vi "New TDMS Property.vi"(8 "error in (no error)":errorcluster, 11 "TDMS Property":T1) -> (0 "error out":errorcluster, 3 "TDMSProperty Ref":T2)   [LabVIEW 2020, in "NI_VS Data Logging API.lvlib"]
doc: "Creates a TdmsProperty object based on the <b>TDMS Property</b> input. The values of TDMS properties that you add to the file, channel groups, or channels, must be scalars of one of the following data types: Timestamp, I8, I16, I32, I64, U8, U16, U32, U64, Single, Double, Boolean, or String. If you set the value to any other data type, or an array of any type, an error will occur."
uses:
  <vilib>/NI VeriStand/Execution/DataLogging/NI_VS Data Logging API.lvlib
  <vilib>/NI VeriStand/Execution/DataLogging/TdmsProperty Ref.ctl
  NationalInstruments.VeriStand.ClientAPI
  <vilib>/NI VeriStand/Execution/DataLogging/TDMS Property.ctl
  <vilib>/NI VeriStand/Execution/DataLogging/Constants.vi
  <vilib>/Utility/VariantDataType/VariantType.lvlib
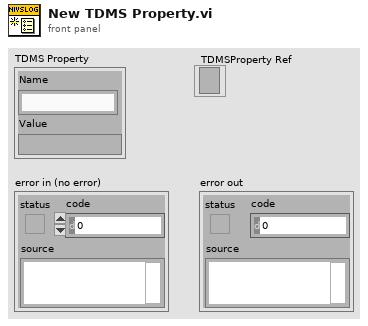
[diagram p1: front panel]
types:
  T1 = typedef "NI_VS Data Logging API.lvlib/TDMS Property.ctl" = cluster{"Name":string, "Value":variant}
  T2 = typedef "NI_VS Data Logging API.lvlib/TdmsProperty Ref.ctl" = refnum<k24>
  T3 = typedef "VariantType.lvlib/Type.ctl" = enum8{"Invalid Type", "Void", "I8", "I16", "I32", "I64", "U8", "U16", "U32", "U64", "Single Float", "Double Float", "Extended Float", "Single Complex", "Double Complex", "Extended Complex", "Enum U8", "Enum U16", "Enum U32", "Enum U64", "Single Float With Unit", "Double Float With Unit", "Extended Float With Unit", "Single Complex with Unit", "Double Complex with Unit", "Extended Complex with Unit", "Boolean", "String", "Path", "Picture", "Tag", "Array", "Cluster", "Variant", "LV Variant", "Waveform", "Timestamp", "Digital Waveform", "Digital Data", "ExpressData", "Refnum", "External Data", "VI", "Poly VI", "LabVIEW Class Instance", "Fixed Point"}
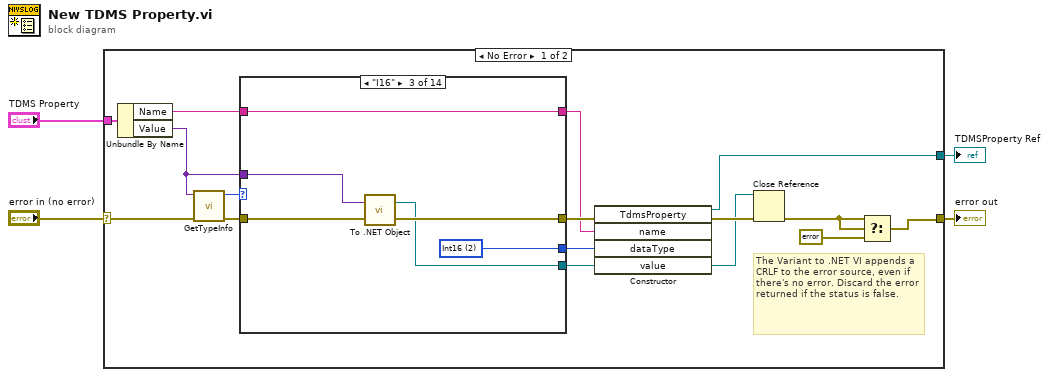
[diagram p0: block diagram]
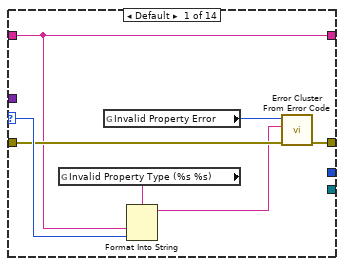
[diagram p2: hidden frame]
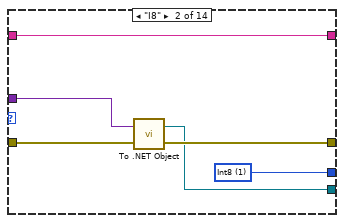
[diagram p3: hidden frame]
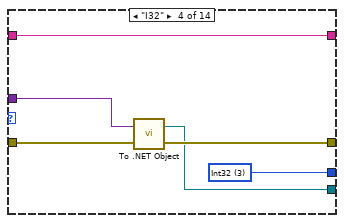
[diagram p4: hidden frame]
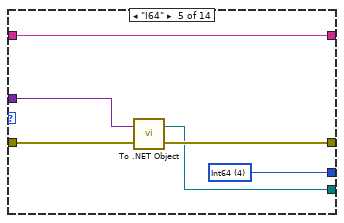
[diagram p5: hidden frame]
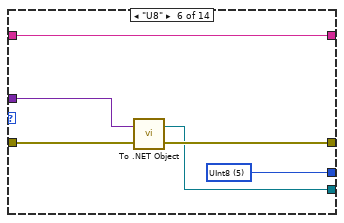
[diagram p6: hidden frame]
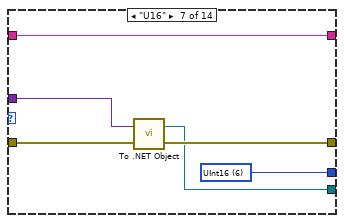
[diagram p7: hidden frame]
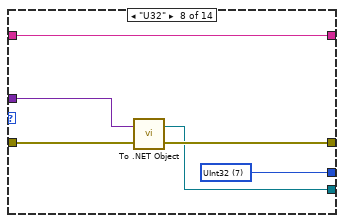
[diagram p8: hidden frame]
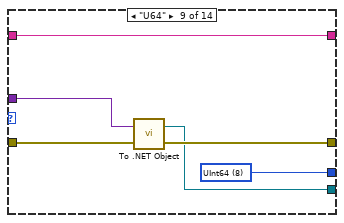
[diagram p9: hidden frame]
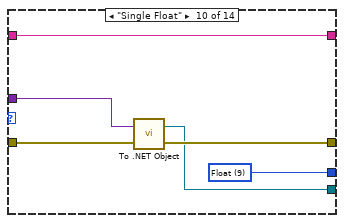
[diagram p10: hidden frame]
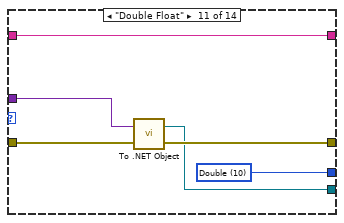
[diagram p11: hidden frame]
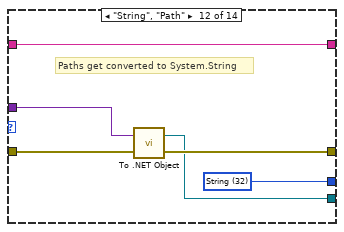
[diagram p12: hidden frame]
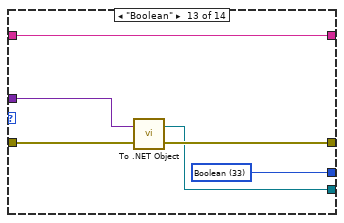
[diagram p13: hidden frame]
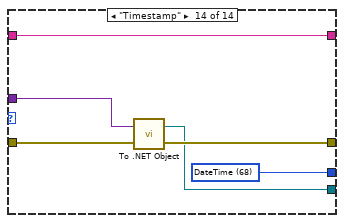
[diagram p14: hidden frame]
diagram:
  n1 = case shown="No Error" "error in (no error)" {
    selector: "error in (no error)" -> [w12 w105]
    tunnel: [w5 w105] -> w4
    tunnel: [w18 _] -> w3
    tunnel: "TDMS Property" -> [w13 _]
    frame No Error {
      # "The Variant to .NET VI appends a CRLF to the error source, even if there's no error. Discard the error returned if the status is false."
      n2 = Unbundle By Name(w13) -> ("Name"=w8:string, "Value"=w16:variant)
      n3 = call <vilib>:"GetTypeInfo.vi"("error in (no error)"=w12, "Variant"=w16) -> ("error out"=w15:errorcluster, "Type Enum"=w14:T3)  [unwired: 5 in, 3 out]
      n4 = case shown="\"I16\"" w14 {
        selector: w14 -> [w26 _ _ _ _ _ _ _ _ _ _ _ _ _]
        tunnel: w15 -> [w25 w31 w37 w43 w49 w55 w61 w67 w73 w79 w85 w91 w97 w103]
        tunnel: w16 -> [_ w30 w36 w42 w48 w54 w60 w66 w72 w78 w84 w90 w96 w102]
        tunnel: [_ w32 w38 w44 w50 w56 w62 w68 w74 w80 w86 w92 w98 w104] -> w17
        tunnel: [w24 w29 w35 w41 w47 w53 w59 w65 w71 w77 w83 w89 w95 w101] -> w19
        tunnel: [_ w28 w34 w40 w46 w52 w58 w64 w70 w76 w82 w88 w94 w100] -> w10
        tunnel: [w20 w27 w33 w39 w45 w51 w57 w63 w69 w75 w81 w87 w93 w99] -> w9
        tunnel: w8 -> [w20 w27 w33 w39 w45 w51 w57 w63 w69 w75 w81 w87 w93 w99]
        frame Default {
          n5 = global read "Constants.vi" "Invalid Property Type (%s %s)"() -> (w23:string)
          n6 = global read "Constants.vi" "Invalid Property Error"() -> (w21:i32)
          n7 = Format Into String(format string=w23, w20, w26) -> (resulting string=w22:string)  [unwired: 2 in, 1 out]
          n8 = call <vilib>:"Error Cluster From Error Code.vi"("error in (no error)"=w25, "error message (\"\")"=w22, "error code (0)"=w21) -> ("error out"=w24:errorcluster)  [unwired: 6 in]
        }
        frame "I8" {
          w32 = 1 items=["Int8"=1, "Int16"=2, "Int32"=3, "Int64"=4, "UInt8"=5, "UInt16"=6, "UInt32"=7, "UInt64"=8, "Float"=9, "Double"=10, "String"=32, "Boolean"=33, "DateTime"=68] ("dataType")
          n9 = call <vilib>:"To .NET Object.vi"("error in (no error)"=w31, "anything"=w30) -> ("error out"=w29:errorcluster, ".NET object"=w28:refnum<k24>)
        }
        frame "I16" {
          w38 = 2 items=["Int8"=1, "Int16"=2, "Int32"=3, "Int64"=4, "UInt8"=5, "UInt16"=6, "UInt32"=7, "UInt64"=8, "Float"=9, "Double"=10, "String"=32, "Boolean"=33, "DateTime"=68] ("dataType")
          n10 = call <vilib>:"To .NET Object.vi"("error in (no error)"=w37, "anything"=w36) -> ("error out"=w35:errorcluster, ".NET object"=w34:refnum<k24>)
        }
        frame "I32" {
          w44 = 3 items=["Int8"=1, "Int16"=2, "Int32"=3, "Int64"=4, "UInt8"=5, "UInt16"=6, "UInt32"=7, "UInt64"=8, "Float"=9, "Double"=10, "String"=32, "Boolean"=33, "DateTime"=68] ("dataType")
          n11 = call <vilib>:"To .NET Object.vi"("error in (no error)"=w43, "anything"=w42) -> ("error out"=w41:errorcluster, ".NET object"=w40:refnum<k24>)
        }
        frame "I64" {
          w50 = 4 items=["Int8"=1, "Int16"=2, "Int32"=3, "Int64"=4, "UInt8"=5, "UInt16"=6, "UInt32"=7, "UInt64"=8, "Float"=9, "Double"=10, "String"=32, "Boolean"=33, "DateTime"=68] ("dataType")
          n12 = call <vilib>:"To .NET Object.vi"("error in (no error)"=w49, "anything"=w48) -> ("error out"=w47:errorcluster, ".NET object"=w46:refnum<k24>)
        }
        frame "U8" {
          w56 = 5 items=["Int8"=1, "Int16"=2, "Int32"=3, "Int64"=4, "UInt8"=5, "UInt16"=6, "UInt32"=7, "UInt64"=8, "Float"=9, "Double"=10, "String"=32, "Boolean"=33, "DateTime"=68] ("dataType")
          n13 = call <vilib>:"To .NET Object.vi"("error in (no error)"=w55, "anything"=w54) -> ("error out"=w53:errorcluster, ".NET object"=w52:refnum<k24>)
        }
        frame "U16" {
          w62 = 6 items=["Int8"=1, "Int16"=2, "Int32"=3, "Int64"=4, "UInt8"=5, "UInt16"=6, "UInt32"=7, "UInt64"=8, "Float"=9, "Double"=10, "String"=32, "Boolean"=33, "DateTime"=68] ("dataType")
          n14 = call <vilib>:"To .NET Object.vi"("error in (no error)"=w61, "anything"=w60) -> ("error out"=w59:errorcluster, ".NET object"=w58:refnum<k24>)
        }
        frame "U32" {
          w68 = 7 items=["Int8"=1, "Int16"=2, "Int32"=3, "Int64"=4, "UInt8"=5, "UInt16"=6, "UInt32"=7, "UInt64"=8, "Float"=9, "Double"=10, "String"=32, "Boolean"=33, "DateTime"=68] ("dataType")
          n15 = call <vilib>:"To .NET Object.vi"("error in (no error)"=w67, "anything"=w66) -> ("error out"=w65:errorcluster, ".NET object"=w64:refnum<k24>)
        }
        frame "U64" {
          w74 = 8 items=["Int8"=1, "Int16"=2, "Int32"=3, "Int64"=4, "UInt8"=5, "UInt16"=6, "UInt32"=7, "UInt64"=8, "Float"=9, "Double"=10, "String"=32, "Boolean"=33, "DateTime"=68] ("dataType")
          n16 = call <vilib>:"To .NET Object.vi"("error in (no error)"=w73, "anything"=w72) -> ("error out"=w71:errorcluster, ".NET object"=w70:refnum<k24>)
        }
        frame "Single Float" {
          w80 = 9 items=["Int8"=1, "Int16"=2, "Int32"=3, "Int64"=4, "UInt8"=5, "UInt16"=6, "UInt32"=7, "UInt64"=8, "Float"=9, "Double"=10, "String"=32, "Boolean"=33, "DateTime"=68] ("dataType")
          n17 = call <vilib>:"To .NET Object.vi"("error in (no error)"=w79, "anything"=w78) -> ("error out"=w77:errorcluster, ".NET object"=w76:refnum<k24>)
        }
        frame "Double Float" {
          w86 = 10 items=["Int8"=1, "Int16"=2, "Int32"=3, "Int64"=4, "UInt8"=5, "UInt16"=6, "UInt32"=7, "UInt64"=8, "Float"=9, "Double"=10, "String"=32, "Boolean"=33, "DateTime"=68] ("dataType")
          n18 = call <vilib>:"To .NET Object.vi"("error in (no error)"=w85, "anything"=w84) -> ("error out"=w83:errorcluster, ".NET object"=w82:refnum<k24>)
        }
        frame "String", "Path" {
          w92 = 32 items=["Int8"=1, "Int16"=2, "Int32"=3, "Int64"=4, "UInt8"=5, "UInt16"=6, "UInt32"=7, "UInt64"=8, "Float"=9, "Double"=10, "String"=32, "Boolean"=33, "DateTime"=68] ("dataType")
          # "Paths get converted to System.String"
          n19 = call <vilib>:"To .NET Object.vi"("error in (no error)"=w91, "anything"=w90) -> ("error out"=w89:errorcluster, ".NET object"=w88:refnum<k24>)
        }
        frame "Boolean" {
          w98 = 33 items=["Int8"=1, "Int16"=2, "Int32"=3, "Int64"=4, "UInt8"=5, "UInt16"=6, "UInt32"=7, "UInt64"=8, "Float"=9, "Double"=10, "String"=32, "Boolean"=33, "DateTime"=68] ("dataType")
          n20 = call <vilib>:"To .NET Object.vi"("error in (no error)"=w97, "anything"=w96) -> ("error out"=w95:errorcluster, ".NET object"=w94:refnum<k24>)
        }
        frame "Timestamp" {
          w104 = 68 items=["Int8"=1, "Int16"=2, "Int32"=3, "Int64"=4, "UInt8"=5, "UInt16"=6, "UInt32"=7, "UInt64"=8, "Float"=9, "Double"=10, "String"=32, "Boolean"=33, "DateTime"=68] ("dataType")
          n21 = call <vilib>:"To .NET Object.vi"("error in (no error)"=w103, "anything"=w102) -> ("error out"=w101:errorcluster, ".NET object"=w100:refnum<k24>)
        }
      }
      n22 = constructor class="TdmsProperty"(error in=w19, "name"=w9, "dataType"=w17, "value"=w10) -> (reference out=w18:refnum<k24>, error out=w11:errorcluster)  [unwired: 2 in, 4 out]
      n23 = Close Reference(reference=w10, error in (no error)=w11) -> (error out=w7:errorcluster)
      n24 = Select(t=w7, s=w7, f=errorcluster {"status"=FALSE, "code"=0, "source"=""}) -> (s? t:f=w5:errorcluster)
    }
    frame Error {
    }
  }
  "error out" <- w4
  "TDMSProperty Ref" <- w3
